vi "Read Tree Ref.vi"(11 "Test Executive Builder View in":refnum<class "Test Executive Builder View.lvclass">) -> (2 "Tree Ref":refnum<vi>, 3 "Test Executive Builder View out":refnum<class "Test Executive Builder View.lvclass">)   [LabVIEW 2017, in "Test Executive Builder View.lvclass"]
uses:
  <vilib>/gpm_packages/@cs/Test-executive-builder/Source/Test Executive Builder View/Test Executive Builder View/Test Executive Builder View.lvclass
  <vilib>/gpm_packages/@cs/Test-executive-builder/Source/Test Executive Builder View/Test Executive Builder View/Test Executive Builder View.lvclass/Test Executive Builder View.ctl
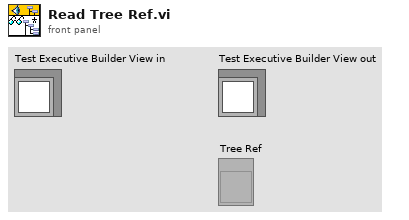
[diagram p1: front panel]
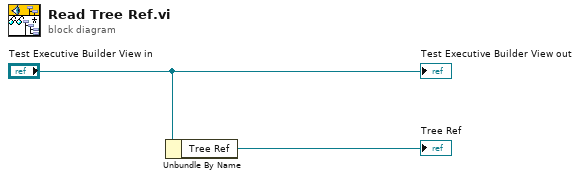
[diagram p0: block diagram]
diagram:
  n1 = Unbundle By Name("Test Executive Builder View in") -> ("Tree Ref"=→"Tree Ref":refnum<vi>)
  "Test Executive Builder View out" <- "Test Executive Builder View in"
